vi "meTEC_Determine List of COM Ports.vi"(8 "error in (no error)":errorcluster) -> (0 "error out":errorcluster, 3 "VISA Resources List (COM Ports)":string[](array[string]))   [LabVIEW 2023]
panel:
  out "Interface Instrument Name List (only for Reference)":string[](array[string])
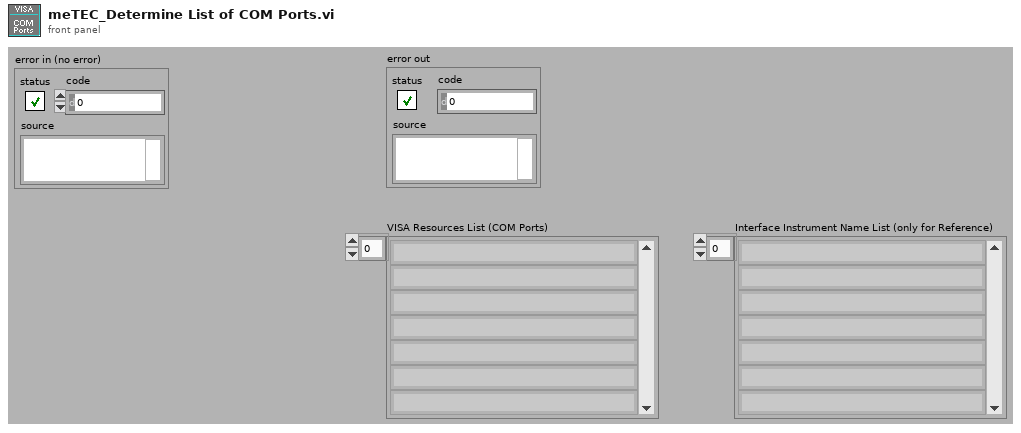
[diagram p1: front panel]
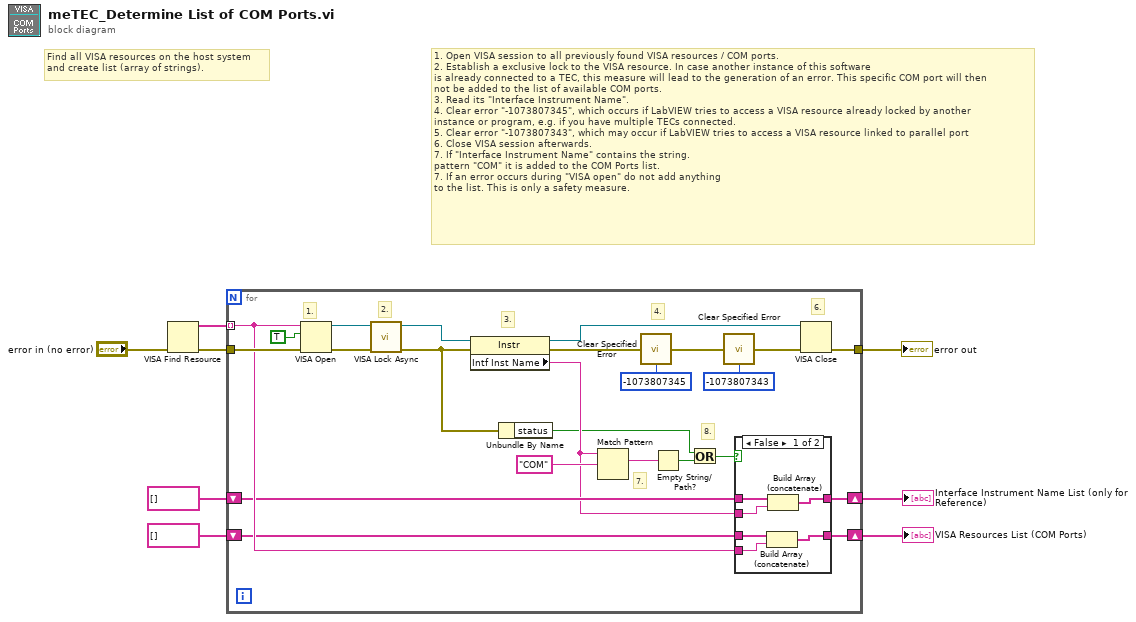
[diagram p0: block diagram]
diagram:
  # "1. Open VISA session to all previously found VISA resources / COM ports.\n2. Establish a exclusive lock to the VISA resource. In case another instance of this software\nis already connected to a TEC, this measure will lead to the generation of an error. This specific COM port will then\nnot be added to the list of available COM ports.\n3. Read its \"Interface Instrument Name\".\n4. Clear error \"-1073807345\", which occurs if LabVIEW tries to access a VISA resource already locked by another \ninstance or program, e.g. if you have multiple TECs connected.\n5. Clear error \"-1073807343\", which may occur if LabVIEW tries to access a VISA resource linked to parallel port\n6. Close VISA session afterwards.\n7. If \"Interface Instrument Name\" contains the string.\npattern \"COM\" it is added to the COM Ports list.\n7. If an error occurs during \"VISA open\" do not add anything\nto the list. This is only a safety measure."
  # "Find all VISA resources on the host system\nand create list (array of strings)."
  n1 = VISA Find Resource(8:"error in (no error)") -> (0:w7:errorcluster, 3:w6:string[])  [unwired: 2 in, 1 out]
  n2 = for {
    tunnel: [w30] -> w4
    tunnel: w7 -> [w32]
    tunnel: w6 -> [w27] mode=indexing
    shift-right: [w26] -> w3
    shift-left: string[] [] -> [w25]
    shift-right: [w23] -> w1
    shift-left: string[] [] -> [w22]
    # "4."
    # "8."
    # "7."
    # "6."
    # "3."
    # "2."
    # "1."
    n3 = VISA Open(duplicate session (F)=TRUE, error in (no error)=w32, VISA resource name=w27) -> (VISA resource name=w14:refnum<visa-resource-name>, error out=w20:errorcluster)  [unwired: 2 in]
    n4 = call <vilib>:"VISA Lock Async.vi"("error in (no error)"=w20, "VISA resource name"=w14) -> ("error out"=w15:errorcluster, "VISA resource name out"=w13:refnum<visa-resource-name>)  [unwired: 7 in, 1 out]
    n5 = property class="Instr"(reference=w13, error in=w15) -> (reference out=w29:refnum<visa-resource-name>, error out=w31:errorcluster, "Intf Inst Name"=w21:string)
    n6 = Unbundle By Name(w15) -> ("status"=w17:bool)
    n7 = Match Pattern(string=w21, regular expression="COM") -> (match substring=w24:string)  [unwired: 1 in, 3 out]
    n8 = call "Clear Specified Error.vi"("error in (no error)"=w31, "Code to Clear (0)"=-1073807345) -> ("error out"=w10:errorcluster)
    n9 = Empty String/Path?(string/path=w24) -> (empty?=w19:bool)
    n10 = Or(x=w17, y=w19) -> (x .or. y?=w18:bool)
    n11 = call "Clear Specified Error.vi"("error in (no error)"=w10, "Code to Clear (0)"=-1073807343) -> ("error out"=w9:errorcluster)
    n12 = case shown="False" w18 {
      tunnel: w27 -> [w38 _]
      tunnel: [w37 w40] -> w26
      tunnel: w25 -> [w36 w40]
      tunnel: w21 -> [w35 _]
      tunnel: [w34 w39] -> w23
      tunnel: w22 -> [w33 w39]
      frame False {
        n13 = Build Array (concatenate)(w36, w38) -> (w37:string[])
        n14 = Build Array (concatenate)(w33, w35) -> (w34:string[])
      }
      frame True {
      }
    }
    n15 = VISA Close(VISA resource name=w29, error in (no error)=w9) -> (error out=w30:errorcluster)
  }
  "error out" <- w4
  "VISA Resources List (COM Ports)" <- w3
  "Interface Instrument Name List (only for Reference)" <- w1
